vi "WS1050_PIC_RFFE_2K_Cycles.vi"(8 "error in (no error)":errorcluster, 9 "Initialize":bool=TRUE, 10 "Number of Cycles":i32=50, 11 "VISA resource name 2":refnum<visa-resource-name>) -> (0 "error out":errorcluster, 2 "No of Cycles Completed":i32, 3 "VISA resource name out":refnum<visa-resource-name>)   [LabVIEW 2009]
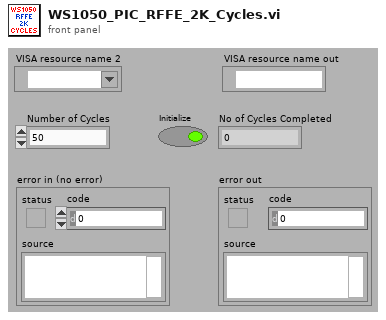
[diagram p1: front panel]
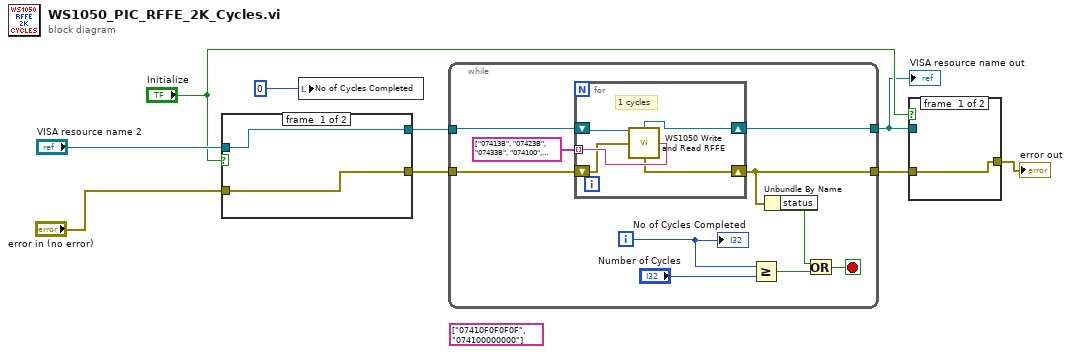
[diagram p0: block diagram]
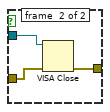
[diagram p2: hidden frame]
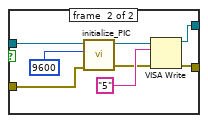
[diagram p3: hidden frame]
diagram:
  (unwired) string[] ["07410F0F0F0F", "074100000000"]
  n1 = case shown="False" "Initialize" {
    tunnel: "error in (no error)" -> [w10 w18]
    tunnel: [w10 w12] -> w8
    tunnel: "VISA resource name 2" -> [w11 w17]
    tunnel: [w11 w13] -> w7
    frame #0 {
    }
    frame #1 {
      n2 = call "initialize_PIC.vi"("error in (no error)"=w18, "baud rate"=u32 9600, "Select Com Port"=w17) -> ("error out"=w15:errorcluster, "VISA resource name out"=w14:refnum<visa-resource-name>)  [unwired: 7 in]
      n3 = VISA Write(VISA resource name=w14, write buffer="5", error in (no error)=w15) -> (VISA resource name out=w13:refnum<visa-resource-name>, error out=w12:errorcluster)  [unwired: 1 out]
    }
  }
  n4 = local write "No of Cycles Completed"(0 ("No of Cycles Completed")) -> ()
  n5 = while {
    tunnel: w8 -> [w29]
    tunnel: w7 -> [w28]
    tunnel: [w27] -> w1
    tunnel: [w26] -> w3
    i -> [w25]
    stop <- w23 stop-if-true
    n6 = for {
      tunnel: string[] ["07413B", "07423B", "07433B", "074100", "074200", "074300"] -> [w34] mode=indexing
      shift-right: [w32] -> w26
      shift-left: w29 -> [w33]
      shift-right: [w31] -> w27
      shift-left: w28 -> [w30]
      # "1 cycles"
      n7 = call "WS1050 Write and Read RFFE.vi"("VISA resource name"=w30, "error in (no error)"=w33, "string to write"=w34) -> ("VISA resource name out"=w31:refnum<visa-resource-name>, "error out"=w32:errorcluster)  [unwired: 8 in, 3 out]
    }
    n8 = Greater Or Equal?(x=w25, y="Number of Cycles") -> (x >= y?=w21:bool)
    n9 = Unbundle By Name(w26) -> ("status"=w22:bool)
    n10 = Or(x=w22, y=w21) -> (x .or. y?=w23:bool)
    "No of Cycles Completed" <- w25
  }
  "VISA resource name out" <- w1
  n11 = case shown="False" "Initialize" {
    tunnel: w1 -> [_ w38]
    tunnel: w3 -> [w35 w37]
    tunnel: [w35 w36] -> w2
    frame #0 {
    }
    frame #1 {
      n12 = VISA Close(VISA resource name=w38, error in (no error)=w37) -> (error out=w36:errorcluster)
    }
  }
  "error out" <- w2
